vi "Folder VI Properties.vi"() -> ()   [LabVIEW 2021]
uses:
  Sub Controls/VI Properties.ctl
panel:
  out "VI Properties":T1[](array[typedef])
  out "All VIs":i32
  out "All Files":i32
  out "Current File":i32
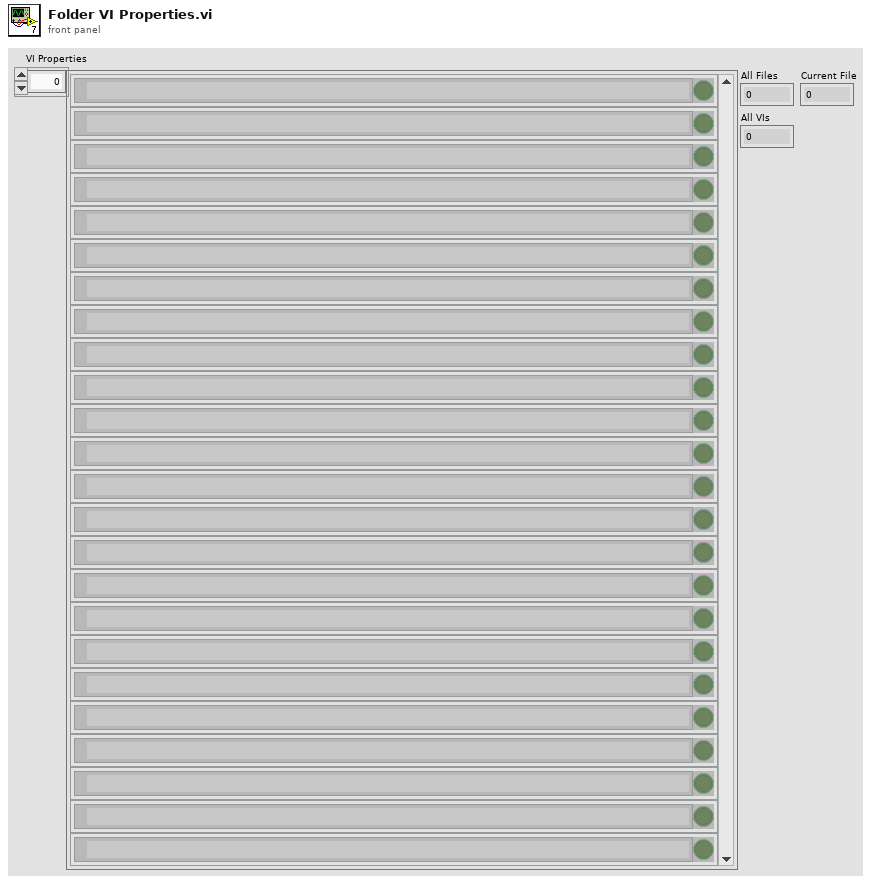
[diagram p1: front panel]
types:
  T1 = typedef "VI Properties.ctl" = cluster{"Reentrant":bool, "Short Path":path, "Full Path":path}
  T2 = enum32{"invalid VI type", "Standard VI", "Control VI", "Global VI", "Polymorphic VI", "Configuration VI", "SubSystem", "Facade VI", "Method VI", "Statechart Diagram VI"}
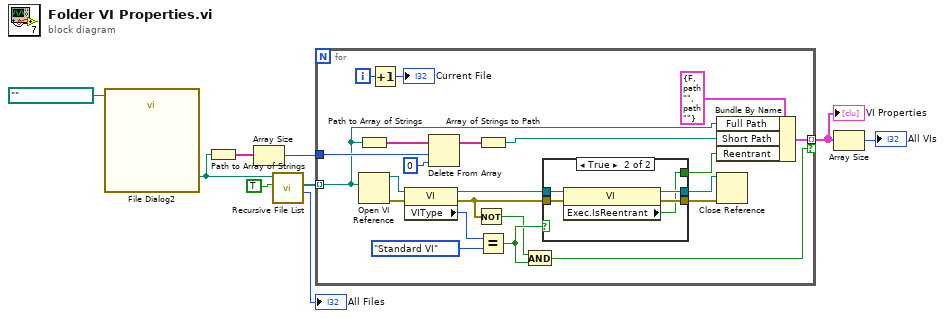
[diagram p0: block diagram]
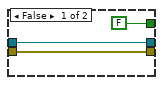
[diagram p2: hidden frame]
diagram:
  n1 = call "File Dialog2"("start path"=path "") -> ("selected path"=w5:path)  [unwired: 11 in, 3 out]
  n2 = Path to Array of Strings(0:w5) -> (2:w7:string[])  [unwired: 1 out]
  n3 = Array Size(array=w7) -> (size(s)=w6:i32)
  n4 = call <vilib>:"Recursive File List.vi"("Treat LLBs as Folders?"=TRUE, "Folder Path"=w5) -> ("Number of Files"=→"All Files":i32, "All Files in Dir"=w4:path[])  [unwired: 5 in, 3 out]
  n5 = for {
    tunnel: w4 -> [w23] mode=indexing
    tunnel: w6 -> [w30]
    tunnel: [w21] -> w2 mode=indexing if=w13
    i -> [w27]
    n6 = Path to Array of Strings(0:w23) -> (2:w31:string[])  [unwired: 1 out]
    n7 = Open VI Reference(vi path=w23) -> (vi reference=w20:refnum<vi>, error out=w17:errorcluster)  [unwired: 5 in]
    n8 = Increment(x=w27) -> (x+1=→"Current File":i32)
    n9 = property class="VI"(reference=w20, error in=w17) -> (reference out=w16:refnum<vi>, error out=w12:errorcluster, "VIType"=w18:T2)
    n10 = Delete From Array(array=w31, length=w30, index=0) -> (array with subset deleted=w29:string[])  [unwired: 1 out]
    n11 = Not(x=w12) -> (.not. x?=w11:bool)
    n12 = Array of Strings to Path(0:w29) -> (2:w22:path)  [unwired: 1 in]
    n13 = Equal?(x=w18, y=T2."Standard VI" ("VI Type")) -> (x = y?=w26:bool)
    n14 = And(x=w11, y=w26) -> (x .and. y?=w13:bool)
    n15 = case shown="True" w26 {
      tunnel: w16 -> [w33 w39]
      tunnel: w12 -> [w34 w38]
      tunnel: [w33 w37] -> w15
      tunnel: [w34 w36] -> w14
      tunnel: [FALSE ("Exec.IsReentrant") w35] -> w24
      frame False {
      }
      frame True {
        n16 = property class="VI"(reference=w39, error in=w38) -> (reference out=w37:refnum<vi>, error out=w36:errorcluster, "Exec.IsReentrant"=w35:bool)
      }
    }
    n17 = Bundle By Name(cluster=T1 {"Reentrant"=FALSE, "Short Path"=path "", "Full Path"=path ""} ("VI Properties"), "Full Path"=w23, "Short Path"=w22, "Reentrant"=w24) -> (w21:T1)
    n18 = Close Reference(reference=w15, error in (no error)=w14) -> ()  [unwired: 1 out]
  }
  "VI Properties" <- w2
  n19 = Array Size(array=w2) -> (size(s)=→"All VIs":i32)
